vi "simulate_mote.vi"() -> ()   [LabVIEW 2011]
uses:
  <vilib>/Platform/TimedLoop/XDataNode/timing_clust.ctl
  <vilib>/Platform/TimedLoop/XDataNode/nitl_modes.ctl
  <vilib>/Platform/TimedLoop/XDataNode/wakeup.ctl
  <vilib>/Platform/TimedLoop/XDataNode/XDataNode.xnode
  <vilib>/Platform/TimedLoop/XDataNode/XDNodeRunTimeDep.lvlib
panel:
  out "element":cluster{string, string, dbl, string, string}
  out "Sending Error":errorcluster
  in  "stop 2":bool
  out "que error":errorcluster
  out "deque error":errorcluster
  in  "stop":bool
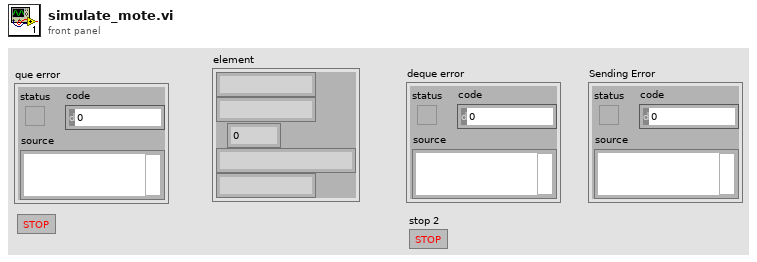
[diagram p1: front panel]
types:
  T1 = enum16{"Read", "Write", "ReadWrite", "BufferedRead", "BufferedReadWrite"}
  T2 = typedef "XDNodeRunTimeDep.lvlib/timing_clust.ctl" = cluster{"Expected End [f-1]":u64, "Actual End [f-1]":u64, "Finished Late? [f-1]":bool, "Expected End [i-1]":u64, "Actual End [i-1]":u64, "Finished Late? [i-1]":bool, "Expected Start [i]":u64, "Actual Start [i]":u64, "Expected Start [f]":u64, "Actual Start [f]":u64, "Source Name":string, "Structure Name":string, "Period":i64, "Deadline":i64, "Offset":i64, "Start":i64, "Priority":i32, "Timeout":i32, "Mode":T3, "Wakeup Reason":T4, "Error":errorcluster, "Source Type":string, "Secondary Source Type":string, "Global End Time":u64, "Global Start Time":u64, "Frame Duration":u64, "Iteration Duration":u64, "Assigned CPU":i32, "I/O Scan Engine Mode":u32}
  T3 = typedef "XDNodeRunTimeDep.lvlib/nitl_modes.ctl" = enum32{"No Change", "Process missed periods, maintain original phase", "Discard missed periods, maintain original phase", "Process missed periods, ignore original phase", "Discard missed periods, ignore original phase"}
  T4 = typedef "XDNodeRunTimeDep.lvlib/wakeup.ctl" = enum32{"Normal", "Aborted", "Asynchronous wakeup", "Timing source error", "Timed loop error", "Timeout"}
  T5 = cluster{string, string, i8, "date/time string":string, string}
  T6 = cluster{string, string, i16, "date/time string":string, string}
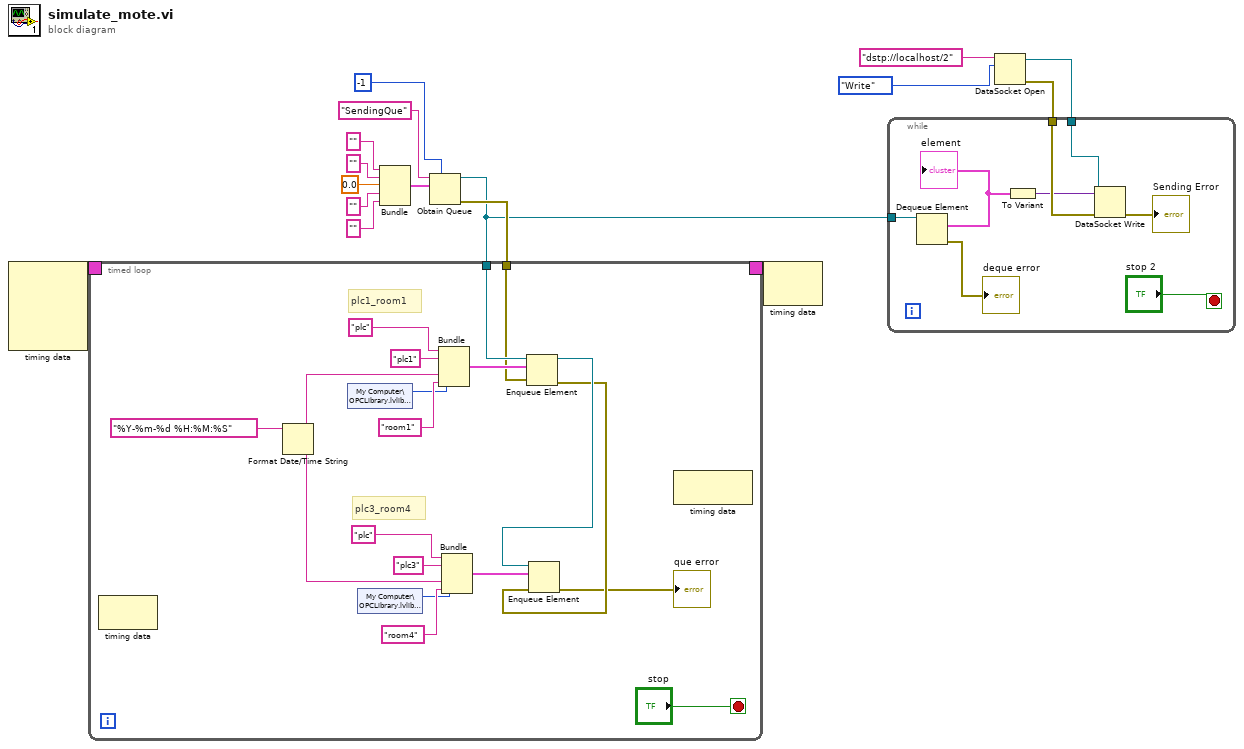
[diagram p0: block diagram]
diagram:
  n1 = node-c288() -> (w16:T2)  [unwired: 4 in]
  n2 = Bundle("", "", 0.0, "", "") -> (w13:cluster{string, string, dbl, string, string})  [unwired: 1 in]
  n3 = Obtain Queue(max queue size (-1, unlimited)=-1, name (unnamed)="SendingQue", element data type=w13) -> (queue out=w5:refnum<queue>, error out=w6:errorcluster)  [unwired: 2 in, 1 out]
  n4 = timed-loop {
    timing: w16 -> [_]
    timing-out: [_] -> w15
    tunnel: w5 -> [w25]
    tunnel: w6 -> [w23]
    stop <- "stop" stop-if-true
    # "plc3_room4"
    # "plc1_room1"
    n5 = node-c288() -> ()  [unwired: 1 in, 1 out]
    n6 = Format Date/Time String(time format string (%c)="%Y-%m-%d %H:%M:%S") -> (date/time string=w19:string)  [unwired: 2 in]
    n7 = shared-variable "My Computer\\OPCLibrary.lvlib\\Int1"() -> (w18:i8)  [unwired: 1 in, 1 out]
    n8 = shared-variable "My Computer\\OPCLibrary.lvlib\\Int2"() -> (w17:i16)  [unwired: 1 in, 1 out]
    n9 = Bundle("plc", "plc1", w18, "date/time string"=w19, "room1") -> (w33:T5)  [unwired: 1 in]
    n10 = Bundle("plc", "plc3", w17, "date/time string"=w19, "room4") -> (w29:T6)  [unwired: 1 in]
    n11 = Enqueue Element(queue=w25, element=w33, error in (no error)=w23) -> (queue out=w24:refnum<queue>, error out=w22:errorcluster)  [unwired: 1 in, 1 out]
    n12 = Enqueue Element(queue=w24, element=w29, error in (no error)=w22) -> (error out=→"que error":errorcluster)  [unwired: 1 in, 2 out]
    n13 = node-c288() -> ()  [unwired: 1 in, 1 out]
  }
  n14 = node-c288(w15) -> ()  [unwired: 1 out]
  n15 = DataSocket Open(10:T1."Write" ("mode"), 11:"dstp://localhost/2" ("URL 3")) -> (0:w1:errorcluster, 3:w2:refnum<k13>)  [unwired: 2 in]
  n16 = while {
    tunnel: w5 -> [w43]
    tunnel: w2 -> [w41]
    tunnel: w1 -> [w40]
    stop <- "stop 2" stop-if-true
    n17 = Dequeue Element(queue=w43) -> (element=w37:cluster{string, string, dbl, string, string}, error out=→"deque error":errorcluster)  [unwired: 2 in, 2 out]
    "element" <- w37
    n18 = To Variant(anything=w37) -> (Variant=w38:variant)
    n19 = DataSocket Write(8:w40, 10:w38, 11:w41) -> (0:→"Sending Error":errorcluster)  [unwired: 3 out]
  }
